vi "Mag_Open.vi"(0 "DIO Module":T3, 1 "Gain (Sensor input field range in Gauss)":T1=32 items=["+/- 1.3"=32, "+/-1.9"=64, "+/-2.5"=96, "+/-4.0"=128, "+/-4.7"=160, "+/-5.6"=192, "+/-8.1"=224], 3 "error in (no error)":errorcluster) -> (7 "I2CDevRef":T2 {"Device Address" format="%.0x"}, 10 "error out":errorcluster)   [LabVIEW 2011]
uses:
  <vilib>/Rock Robotics/SystemInterfaces/Typedef/FPGA_TypedefDigitalModule.ctl
  <vilib>/Rock Robotics/WPI/I2C/WPI_I2CDevRef.ctl
  Mag _Gain.ctl
panel:
  in  "CRA_REG_M":u8=28 format="%x"
  # "Use table to the left"
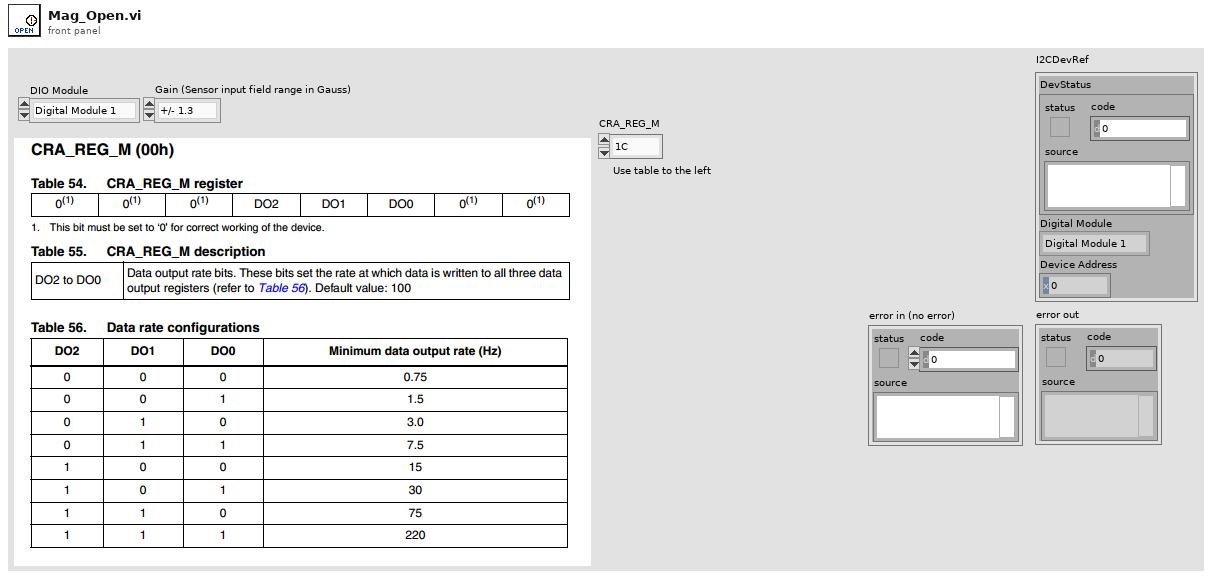
[diagram p1: front panel]
types:
  T1 = typedef "Mag _Gain.ctl" = u8
  T2 = typedef "WPI_I2CDevRef.ctl" = cluster{"DevStatus":errorcluster, "Digital Module":T3, "Device Address":u8}
  T3 = typedef "FPGA_TypedefDigitalModule.ctl" = enum16{"Digital Module 1", "Digital Module 2"}
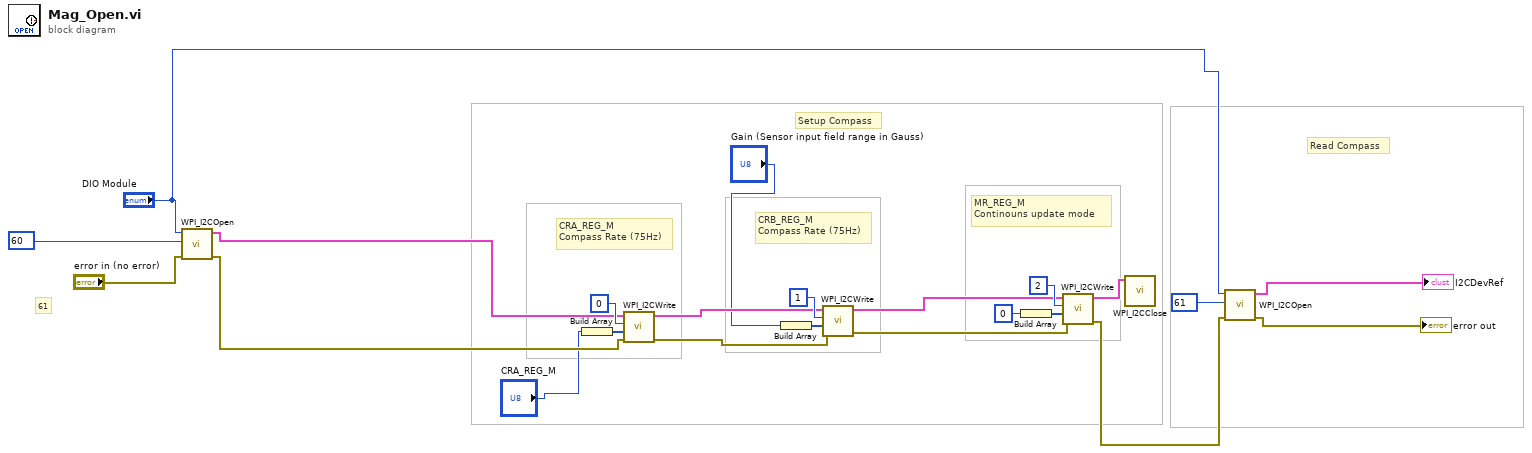
[diagram p0: block diagram]
diagram:
  # "Read Compass"
  # "61"
  # "Setup Compass"
  # "MR_REG_M\nContinouns update mode"
  # "CRB_REG_M\nCompass Rate (75Hz)"
  # "CRA_REG_M\nCompass Rate (75Hz)"
  n1 = call <vilib>:"WPI_I2COpen.vi"("error in (no error)"="error in (no error)", "Device Address"=u8 60 ("Data To Send"), "Digital Module (Module 1)"="DIO Module") -> ("error out"=w9:errorcluster, "I2CDevRef"=w10:T2)  [unwired: 7 out]
  n2 = Build Array("CRA_REG_M") -> (w21:u8[])
  n3 = call <vilib>:"WPI_I2CWrite.vi"("error in (no error)"=w9, "I2CDataToSend"=w21, "I2CRegister"=u8 0 ("Data To Send"), "I2CDevRef"=w10) -> ("error out"=w17:errorcluster, "I2CDevRef"=w18:T2)  [unwired: 1 in, 5 out]
  n4 = Build Array("Gain (Sensor input field range in Gauss)") -> (w19:T1[])
  n5 = call <vilib>:"WPI_I2CWrite.vi"("error in (no error)"=w17, "I2CDataToSend"=w19, "I2CRegister"=u8 1 ("Data To Send"), "I2CDevRef"=w18) -> ("error out"=w12:errorcluster, "I2CDevRef"=w11:T2)  [unwired: 1 in, 5 out]
  n6 = Build Array(u8 0 ("Data To Send")) -> (w13:u8[])
  n7 = call <vilib>:"WPI_I2CWrite.vi"("error in (no error)"=w12, "I2CDataToSend"=w13, "I2CRegister"=u8 2 ("Data To Send"), "I2CDevRef"=w11) -> ("error out"=w4:errorcluster, "I2CDevRef"=w1:T2)  [unwired: 1 in, 5 out]
  n8 = call <vilib>:"WPI_I2CClose.vi"("I2CDevRef"=w1) -> ()  [unwired: 10 in, 1 out]
  n9 = call <vilib>:"WPI_I2COpen.vi"("error in (no error)"=w4, "Device Address"=u8 61 ("Data To Send"), "Digital Module (Module 1)"="DIO Module") -> ("error out"=→"error out":errorcluster, "I2CDevRef"=→"I2CDevRef":T2)  [unwired: 7 out]
